vi "Write Payload.vi"(8 "error in (no error)":errorcluster, 10 "Payload In":refnum<class "RDS Payload.lvclass">, 11 "RDS Message in":refnum<class "RDS Message.lvclass">) -> (0 "error out":errorcluster, 3 "RDS Message out":refnum<class "RDS Message.lvclass">)   [LabVIEW 2015]
uses:
  RDS Message.lvclass
  RDS Payload Class/RDS Payload.lvclass
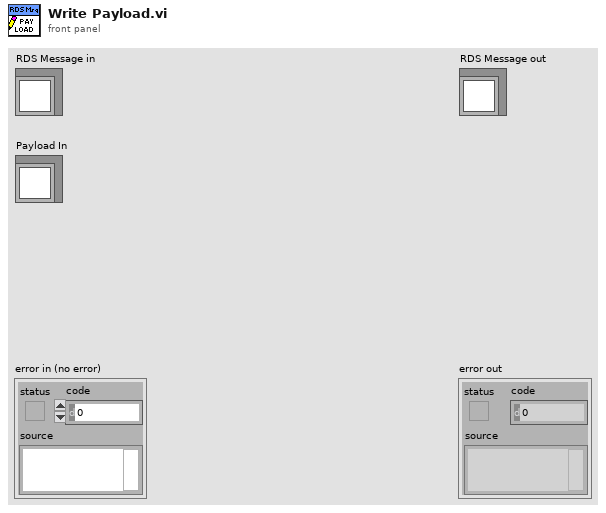
[diagram p1: front panel]
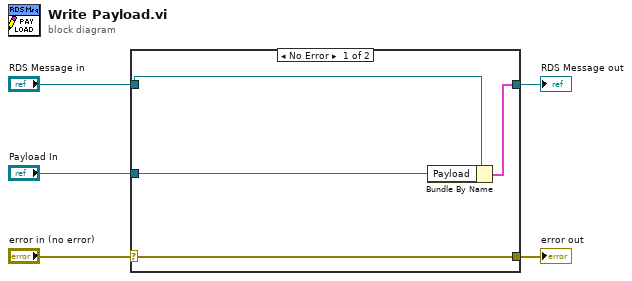
[diagram p0: block diagram]
diagram:
  n1 = case shown="No Error" "error in (no error)" {
    selector: "error in (no error)" -> [w9 w10]
    tunnel: [w9 w10] -> w4
    tunnel: [w7 w11] -> w2
    tunnel: "RDS Message in" -> [w8 w11]
    tunnel: "Payload In" -> [w6 _]
    frame No Error {
      n2 = Bundle By Name(cluster=w8, "Payload"=w6) -> (w7:cluster{})
    }
    frame Error {
    }
  }
  "error out" <- w4
  "RDS Message out" <- w2
